vi "PH_ImageOperator.Target Fnc & Deriv GAUSSs.vi"(0 "Flag":enum16{"no deriv", "deriv"}(ring), 1 "Order of GAUSSian function":i32, 2 "Coefficients":dbl[](array[numeric]) format="%0.5f", 3 "X":dbl format="%0.3f", 4 "No Offset?":bool) -> (5 "Y":dbl format="%0.3f", 6 "Derivatives":dbl[](array[numeric]) format="%0.5f")   [LabVIEW 2014, in "PH_ImageOperator.lvlib"]
doc: "Here the user specifies his guess at the functional form of the relationship between Y and X as a function of coefficients. \n\nIf the partial derivatives of the function are known, the user also furnishes the equations for the partial derivatives of this function with respect to each coefficient. The input control Flag should then be set to 1 (deriv) by all calling VIs.\n\nIf the partial derivatives of the function are not known, the input control Flag should be set to 0 (no deriv) by all calling VIs, and a numerical approximation to the partial derivatives will be computed."
uses:
  PH_ImageOperator.lvlib
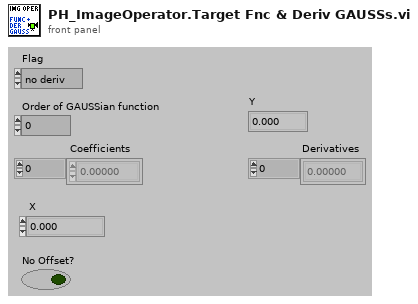
[diagram p1: front panel]
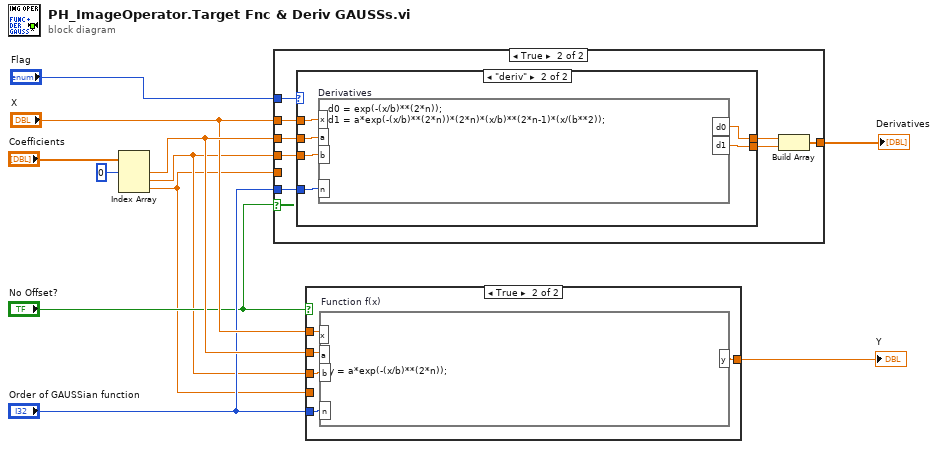
[diagram p0: block diagram]
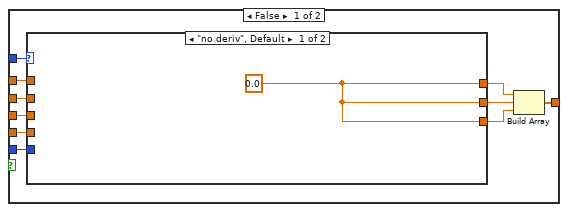
[diagram p2: hidden frame]
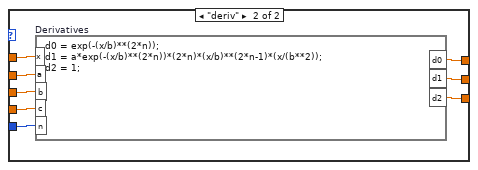
[diagram p3: hidden frame]
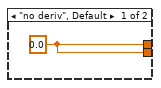
[diagram p4: hidden frame]
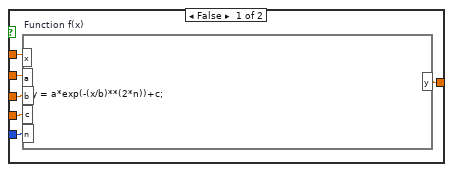
[diagram p5: hidden frame]
diagram:
  n1 = Index Array(array="Coefficients", index #1=0) -> (element #1=w9:dbl, element #2=w2:dbl, element #3=w1:dbl)  [unwired: 2 in]
  n2 = case shown="True" "No Offset?" {
    tunnel: w9 -> [w21 w38]
    tunnel: w2 -> [w20 w37]
    tunnel: w1 -> [w19 _]
    tunnel: "X" -> [w18 w36]
    tunnel: "Order of GAUSSian function" -> [w17 w35]
    tunnel: [w13 w32] -> w3
    tunnel: "Flag" -> [w12 w31]
    frame False {
      n3 = case shown="\"no deriv\", Default" w12 {
        tunnel: w21 -> [_ w30]
        tunnel: w20 -> [_ w29]
        tunnel: w19 -> [_ w28]
        tunnel: w18 -> [_ w27]
        tunnel: w17 -> [_ w26]
        tunnel: [w22 w25] -> w16
        tunnel: [w22 w24] -> w15
        tunnel: [w22 w23] -> w14
        frame "no deriv", Default {
          w22 = 0.0 ("d0")
        }
        frame "deriv" {
          n4 = formula code="d0 = exp(-(x/b)**(2*n));\nd1 = a*exp(-(x/b)**(2*n))*(2*n)*(x/b)**(2*n-1)*(x/(b**2));\nd2 = 1;" "Derivatives"("x"=w27, "a"=w30, "b"=w29, "c"=w28, "n"=w26) -> ("d0"=w23:dbl, "d1"=w24:dbl, "d2"=w25:dbl)
        }
      }
      n5 = Build Array(w14, w15, w16) -> (w13:dbl[])
    }
    frame True {
      n6 = case shown="\"deriv\"" w31 {
        tunnel: w38 -> [_ w45]
        tunnel: w37 -> [_ w44]
        tunnel: w36 -> [_ w43]
        tunnel: w35 -> [_ w42]
        tunnel: [w39 w41] -> w34
        tunnel: [w39 w40] -> w33
        frame "no deriv", Default {
          w39 = 0.0 ("d0")
        }
        frame "deriv" {
          n7 = formula code="d0 = exp(-(x/b)**(2*n));\nd1 = a*exp(-(x/b)**(2*n))*(2*n)*(x/b)**(2*n-1)*(x/(b**2));" "Derivatives"("x"=w43, "a"=w45, "b"=w44, "n"=w42) -> ("d0"=w40:dbl, "d1"=w41:dbl)
        }
      }
      n8 = Build Array(w33, w34) -> (w32:dbl[])
    }
  }
  "Derivatives" <- w3
  n9 = case shown="True" "No Offset?" {
    tunnel: [w51 w56] -> w10
    tunnel: w9 -> [w50 w55]
    tunnel: w2 -> [w49 w54]
    tunnel: w1 -> [w48 _]
    tunnel: "X" -> [w47 w53]
    tunnel: "Order of GAUSSian function" -> [w46 w52]
    frame False {
      n10 = formula code="y = a*exp(-(x/b)**(2*n))+c;" "Function f(x)"("x"=w47, "a"=w50, "b"=w49, "c"=w48, "n"=w46) -> ("y"=w51:dbl)
    }
    frame True {
      n11 = formula code="y = a*exp(-(x/b)**(2*n));" "Function f(x)"("x"=w53, "a"=w55, "b"=w54, "n"=w52) -> ("y"=w56:dbl)
    }
  }
  "Y" <- w10
